vi "getData.vi"(8 "error in (no error)":errorcluster, 11 "RampEvent in":refnum<class "RampEvent.lvclass">) -> (0 "error out":errorcluster, 1 "dataType":T1(ring), 2 "data":T2, 3 "RampEvent out":refnum<class "RampEvent.lvclass">)   [LabVIEW 2009, in "Tools.lvlib" / "Scripting.lvlib" / "RampEvent.lvclass"]
uses:
  RampEvent.lvclass
  DatabaseHelpers/Database Objects/Channel/Channel.lvclass
  RampEvent.lvclass/RampEvent.ctl
  ScriptEvent.lvclass
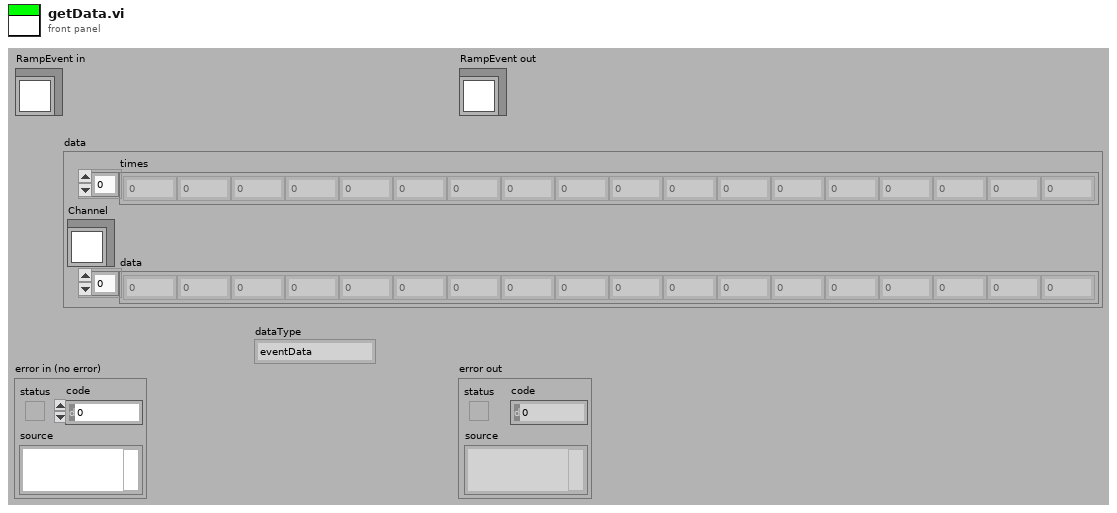
[diagram p1: front panel]
types:
  T1 = enum16{"eventData", "singleToneData", "fileData"}
  T2 = cluster{"times":dbl[], "Channel":refnum<class "Channel.lvclass">, "data":dbl[]}
  T3 = cluster{dbl[], "Channel.lvclass":refnum<class "Channel.lvclass">, dbl[]}
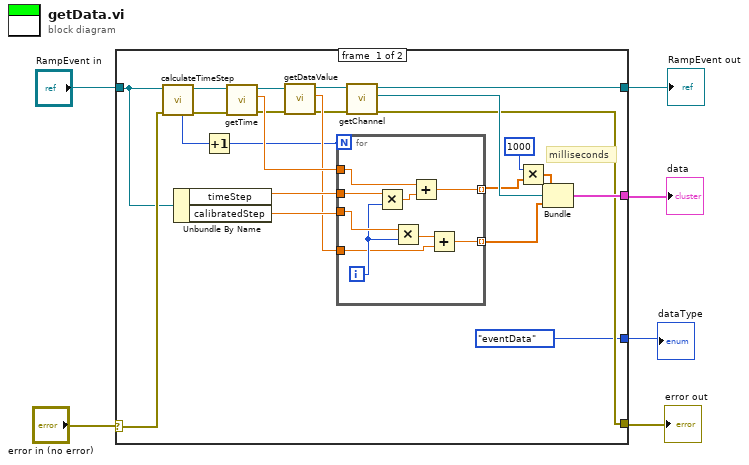
[diagram p0: block diagram]
diagram:
  n1 = case shown="No Error" "error in (no error)" {
    selector: "error in (no error)" -> [w29 w39]
    tunnel: [w14 w40] -> w6
    tunnel: "RampEvent in" -> [w27 w40]
    tunnel: [w11 w39] -> w3
    tunnel: [w15 _] -> w2
    tunnel: [T1."eventData" ("dataType") _] -> w1
    frame #0 {
      # "milliseconds"
      n2 = call "calculateTimeStep.vi"("error in (no error)"=w29, "RampEvent in"=w27) -> ("error out"=w25:errorcluster, "RampEvent out"=w26:refnum<class "RampEvent.lvclass">, "number of Steps"=w28:i32)  [unwired: 5 in, 2 out]
      n3 = Unbundle By Name(w27) -> ("timeStep"=w23:dbl, "calibratedStep"=w22:dbl)
      n4 = Increment(x=w28) -> (x+1=w13:i32)
      n5 = call "getTime.vi"("error in (no error)"=w25, "ScriptEvent.lvclass in"=w26) -> ("error out"=w20:errorcluster, "time"=w24:dbl, "ScriptEvent.lvclass out"=w21:refnum<class "RampEvent.lvclass">)  [unwired: 7 in]
      n6 = call "getDataValue.vi"("error in (no error)"=w20, "ScriptEvent.lvclass in"=w21) -> ("error out"=w18:errorcluster, "dataValue"=w19:dbl, "ScriptEvent.lvclass out"=w17:refnum<class "RampEvent.lvclass">)  [unwired: 7 in]
      n7 = for {
        N: w13 -> [_]
        tunnel: w24 -> [w37]
        tunnel: w23 -> [w38]
        tunnel: w22 -> [w35]
        tunnel: w19 -> [w32]
        tunnel: [w31] -> w10 mode=indexing
        tunnel: [w30] -> w16 mode=indexing
        i -> [w34]
        n8 = Multiply(x=w38, y=w34) -> (x*y=w36:dbl)
        n9 = Multiply(x=w35, y=w34) -> (x*y=w33:dbl)
        n10 = Add(x=w37, y=w36) -> (x+y=w31:dbl)
        n11 = Add(x=w33, y=w32) -> (x+y=w30:dbl)
      }
      n12 = call-dynamic "getChannel.vi"("error in (no error)"=w18, "ScriptEvent.lvclass in"=w17) -> ("error out"=w11:errorcluster, "Channel.lvclass"=w12:refnum<class "Channel.lvclass">, "ScriptEvent.lvclass out"=w14:refnum<class "RampEvent.lvclass">)  [unwired: 7 in]
      n13 = Multiply(x=1000, y=w10) -> (x*y=w9:dbl[])
      n14 = Bundle(w9, "Channel.lvclass"=w12, w16) -> (w15:T3)  [unwired: 1 in]
    }
    frame #1 {
    }
  }
  "error out" <- w3
  "RampEvent out" <- w6
  "data" <- w2
  "dataType" <- w1
